vi "Generic IED Test.vi"(8 "error in":errorcluster, 11 "IED Test in":refnum<class "IED Test.lvclass">) -> (0 "error out":errorcluster, 2 "Test Result":T1=enum."Success", 3 "IED Test out":refnum<class "IED Test.lvclass">)   [LabVIEW 2018, in "IED Test Framework.lvlib" / "IED Test.lvclass"]
uses:
  IED Test.lvclass
  C:/Program Files (x86)/National Instruments/LabVIEW 2018/vi.lib/ActorFramework/Actor/Actor.lvclass
  C:/Users/Administrator/Desktop/2018LabVIEW EMS/EMS Generic Actor/EMS Generic/EMS Generic.lvclass
  Controls/Test Result.ctl
  IED Actor/IED/IED.lvclass
  C:/Users/Administrator/Desktop/2018LabVIEW EMS/IED Actors/Device DDS Communications Framework/Device DDS Communications/Device DDS Communications.lvclass
  <vilib>/ORNL/CSEISMIC DDS/CSEISMIC DDS Base/Data Types/Controls/DeviceClass Selector.ctl
  <vilib>/ORNL/CSEISMIC DDS/CSEISMIC DDS Base/CSEISMIC DDS.lvclass/CSEISMIC DDS.ctl
  <vilib>/ActorFramework/Message Enqueuer/Message Enqueuer.lvclass/Message Enqueuer.ctl
  <vilib>/ORNL/CSEISMIC DDS/CSEISMIC DDS Base/Data Types/Controls/DeviceID.ctl
  <vilib>/ORNL/CSEISMIC DDS/CSEISMIC DDS Base/Accessors/Write DDS Reference.vi
  <vilib>/ActorFramework/Message Enqueuer/Enqueue.vi
  <vilib>/ORNL/CSEISMIC DDS/CSEISMIC DDS Base/Accessors/Read DDS Reference.vi
  <vilib>/ORNL/CSEISMIC DDS/DDS Reader/DDS Reader.lvclass
  C:/Program Files (x86)/National Instruments/LabVIEW 2018/vi.lib/ORNL/CSEISMIC DDS/CSEISMIC DDS Base/CSEISMIC DDS.lvclass
  IED Actor/IED Messages/Set Microgrid ID Msg/Set Microgrid ID Msg.lvclass
  C:/Program Files (x86)/National Instruments/LabVIEW 2018/vi.lib/ActorFramework/Message/Message.lvclass
  <vilib>/ORNL/CSEISMIC DDS/DDS Writer/DDS Writer.lvclass
  <vilib>/ActorFramework/Stop Msg/Stop Msg.lvclass
  <vilib>/ORNL/CSEISMIC DDS/CSEISMIC DDS Base/Error Handler.vi
  <vilib>/ActorFramework/Message Priority Queue/Priority Enqueue.vi
  Device DDS Communications Framework/Device DDS Communications/Device DDS Communications.lvclass
  <vilib>/ActorFramework/Actor/Actor.lvclass
  <vilib>/ORNL/CSEISMIC DDS/CSEISMIC DDS Base/CSEISMIC DDS.lvclass
  EMS Generic Actor/EMS Generic/EMS Generic.lvclass
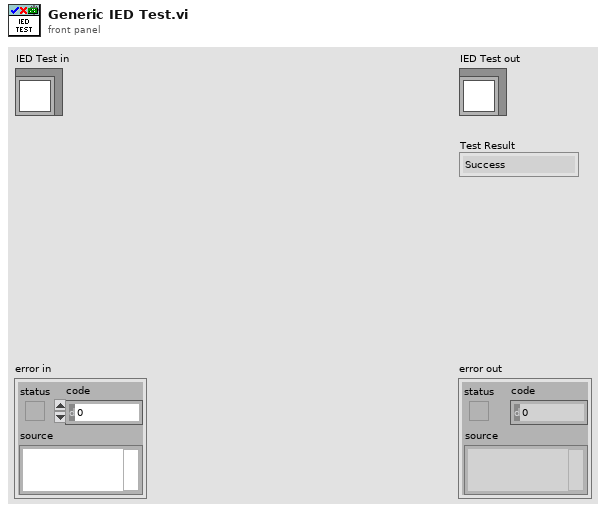
[diagram p1: front panel]
types:
  T1 = typedef "IED Test Framework.lvlib/IED Test.lvclass/Test Result.ctl" = enum16{"Invalid", "Success", "Failure", "Error", "Timeout"}
  T2 = typedef "CSEISMIC DDS.lvlib/CSEISMIC DDS.lvclass/DeviceID.ctl" = string
  T3 = typedef "CSEISMIC DDS.lvlib/CSEISMIC DDS.lvclass/DeviceClass Selector.ctl" = u16
  T4 = typedef "CSEISMIC DDS.lvlib/CSEISMIC DDS.lvclass/IED_setMicrogridID.ctl" = cluster{"DeviceID":T2, "MicrogridID":u8}
  T5 = typedef "CSEISMIC DDS.lvlib/CSEISMIC DDS.lvclass/IED_Status.ctl" = cluster{"DeviceID":T2, "Timestamp":T6, "MicrogridID":u8, "Active":bool, "Inactive":bool, "Error":i32, "Fault":bool, "ErrorString":string}
  T6 = typedef "CSEISMIC DDS.lvlib/CSEISMIC DDS.lvclass/Timestamp.ctl" = cluster{"Seconds":u64, "Remainder":u64}
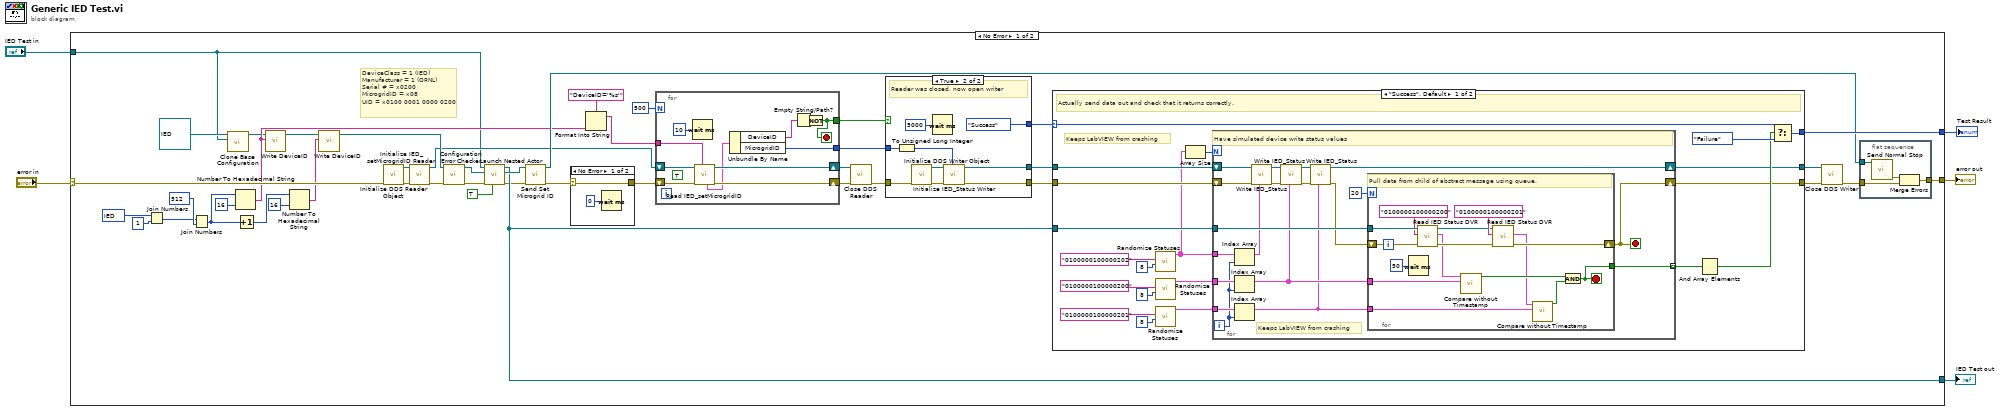
[diagram p0: block diagram]
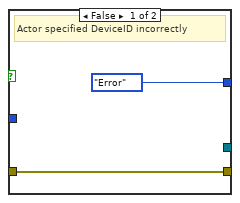
[diagram p3: hidden frame]
diagram:
  n1 = case shown="No Error" "error in" {
    selector: "error in" -> [w27 w138]
    tunnel: [w34 w138] -> w4
    tunnel: [w40 w137] -> w2
    tunnel: "IED Test in" -> [w6 w137]
    tunnel: [w37 _] -> w1
    frame No Error {
      w28 = T3 256 items=["Invalid"=0, "IED"=256, "DER"=512, "Relay"=768, "Meter"=1024, "Load"=1280, "Forecast"=1536, "Price"=1792, "Energy Storage"=513, "PV"=514, "Generator"=515, "Smart Relay"=769, "PCC"=770, "Smart Meter"=1025, "PMU"=1026, "HVAC"=1281] ("DeviceClass")
      # "DeviceClass = 1 (IED)\nManufacturer = 1 (ORNL)\nSerial # = x0200\nMicrogridID = x08\nUID = x0100 0001 0000 0200"
      n2 = Join Numbers(hi=w28, lo=u16 1 ("MicrogridID")) -> ((hi.lo)=w45:u32)
      n3 = Join Numbers(hi=w45, lo=u32 512 ("MicrogridID")) -> ((hi.lo)=w18:u64)
      n4 = call-dynamic "Clone Base Configuration.vi"("Source Object"=w6, "Target Object in"=refnum<class "IED.lvclass"> refnum ("IED Framework.lvlib:IED.lvclass")) -> ("Target Object out"=w7:refnum<class "IED.lvclass">)  [unwired: 9 in]
      n5 = Number To Hexadecimal String(1:i16 16 ("width (-)"), 2:w18) -> (0:w10:string)
      n6 = Increment(x=w18) -> (x+1=w16:u64)
      n7 = call-dynamic "Write DeviceID.vi"("DeviceID"=w10, "Device DDS Communications in"=w7) -> ("Device DDS Communications out"=w36:refnum<class "IED.lvclass">)  [unwired: 9 in]
      n8 = Number To Hexadecimal String(1:i16 16 ("width (-)"), 2:w16) -> (0:w15:string)
      n9 = call-dynamic "Write DeviceID.vi"("DeviceID"=w15, "Device DDS Communications in"=w36) -> ("Device DDS Communications out"=w35:refnum<class "IED.lvclass">)  [unwired: 9 in]
      n10 = call <vilib>:"Initialize DDS Reader Object.vi"("error in"=w27) -> ("error out"=w26:errorcluster, "DDS Reader out"=w25:refnum<class "DDS Reader.lvclass">)  [unwired: 9 in]
      n11 = call <vilib>:"Initialize IED_setMicrogridID Reader.vi"("error in"=w26, "DDS Reader in"=w25) -> ("error out"=w24:errorcluster, "DDS Reader out"=w23:refnum<class "DDS Reader.lvclass">)  [unwired: 8 in]
      n12 = call "Configuration Error Checker.vi"("error in"=w24, "Device DDS Communications in"=w35) -> ("error out"=w48:errorcluster, "Device DDS Communications out"=w47:refnum<class "IED.lvclass">)  [unwired: 8 in]
      n13 = call <vilib>:"Launch Nested Actor.vi"("Open Actor Core front panel? (F)"=TRUE, "error in (no error)"=w48, "Nested Actor"=w47, "Caller Actor in"=w6) -> ("error out"=w31:errorcluster, "Nested Actor's Enqueuer"=w49:refnum<class "Message Enqueuer.lvclass">, "Caller Actor out"=w40:refnum<class "IED Test.lvclass">)  [unwired: 5 in]
      n14 = call "Send Set Microgrid ID.vi"("error in (no error)"=w31, "Message Enqueuer"=w49) -> ("error out"=w30:errorcluster, "Message Enqueuer out"=w33:refnum<class "Message Enqueuer.lvclass">)  [unwired: 8 in]
      n15 = case shown="No Error" w30 {
        selector: w30 -> [w134 w136]
        tunnel: [w134 w136] -> w29
        frame No Error {
          n16 = Wait (ms)(milliseconds to wait=u32 0) -> ()  [unwired: 1 out]
        }
        frame Error {
        }
      }
      n17 = Format Into String(format string="DeviceID='%s'", w10) -> (resulting string=w9:string)  [unwired: 2 in, 1 out]
      n18 = for {
        N: 500 -> [_]
        tunnel: [w122] -> w43
        tunnel: [w118] -> w42
        shift-right: [w114] -> w21
        shift-left: w23 -> [w117]
        shift-right: [w115] -> w22
        shift-left: w29 -> [w116]
        tunnel: w9 -> [w112]
        stop <- w118 stop-if-true
        (unwired) TRUE ("only new samples")
        n19 = Wait (ms)(milliseconds to wait=u32 10) -> ()  [unwired: 1 out]
        n20 = call <vilib>:"Read IED_setMicrogridID.vi"("Query condition"=w112, "error in"=w116, "DDS Reader in"=w117) -> ("error out"=w115:errorcluster, "DDS Reader out"=w114:refnum<class "DDS Reader.lvclass">, "data"=w113:T4)  [unwired: 5 in, 1 out]
        n21 = Unbundle By Name(w113) -> ("DeviceID"=w121:T2, "MicrogridID"=w122:u8)
        n22 = Empty String/Path?(string/path=w121) -> (empty?=w119:bool)
        n23 = Not(x=w119) -> (.not. x?=w118:bool)
      }
      n24 = call <vilib>:"Close DDS Reader.vi"("error in"=w22, "DDS Reader in"=w21) -> ("error out"=w20:errorcluster)  [unwired: 9 in]
      n25 = case shown="True" w42 {
        tunnel: [w124 w128] -> w39
        tunnel: w20 -> [w124 w130]
        tunnel: w43 -> [_ w133]
        tunnel: [_ w125] -> w41
        tunnel: [Test_Result."Error" ("Test Result") Test_Result."Success" ("Test Result")] -> w38
        frame False {
          # "Actor specified DeviceID incorrectly"
        }
        frame True {
          # "Reader was closed, now open writer"
          n26 = To Unsigned Long Integer(number=w133) -> (unsigned 32bit integer=w126:u32)
          n27 = call <vilib>:"Initialize DDS Writer Object.vi"("error in"=w130) -> ("error out"=w129:errorcluster, "DDS Writer out"=w127:refnum<class "DDS Writer.lvclass">)  [unwired: 9 in]
          n28 = Wait (ms)(milliseconds to wait=u32 5000) -> ()  [unwired: 1 out]
          n29 = call <vilib>:"Initialize IED_Status Writer.vi"("MicrogridID"=w126, "error in"=w129, "DDS Writer in"=w127) -> ("error out"=w128:errorcluster, "DDS Writer out"=w125:refnum<class "DDS Writer.lvclass">)  [unwired: 7 in]
        }
      }
      n30 = case shown="\"Success\", Default" w38 {
        selector: w38 -> [w73 w110]
        tunnel: w41 -> [w74 w109]
        tunnel: w40 -> [w60 _]
        tunnel: w39 -> [w61 w111]
        tunnel: [w71 w110] -> w37
        tunnel: [w59 w111] -> w14
        tunnel: [w55 w109] -> w12
        frame "Success", Default {
          # "Keeps LabVIEW from crashing"
          # "Actually send data out and check that it returns correctly."
          n31 = call "Randomize Statuses.vi"("MicrogridID"=u16 8, "DeviceID"=T2 "0100000100000202" ("(hi.lo)")) -> ("IED Status Array out"=w56:T5[])  [unwired: 9 in]
          n32 = call "Randomize Statuses.vi"("MicrogridID"=u16 8, "DeviceID"=T2 "0100000100000200" ("(hi.lo)")) -> ("IED Status Array out"=w62:T5[])  [unwired: 9 in]
          n33 = call "Randomize Statuses.vi"("MicrogridID"=u16 8, "DeviceID"=T2 "0100000100000201" ("(hi.lo)")) -> ("IED Status Array out"=w63:T5[])  [unwired: 9 in]
          n34 = Array Size(array=w56) -> (size(s)=w57:i32)
          n35 = for {
            N: w57 -> [_]
            shift-right: [w90] -> w55
            shift-left: w74 -> [w93]
            tunnel: w56 -> [w86]
            tunnel: w63 -> [w81]
            tunnel: w62 -> [w82]
            shift-right: [w83] -> w59
            shift-left: w61 -> [w89]
            tunnel: w60 -> [w85]
            tunnel: [w75] -> w58 mode=indexing
            i -> [w78]
            stop <- w83 stop-if-true
            # "Keeps LabVIEW from crashing"
            # "Have simulated device write status values"
            n36 = Index Array(array=w86, index=w78) -> (element=w79:T5)
            n37 = Index Array(array=w82, index=w78) -> (element=w77:T5)
            n38 = Index Array(array=w81, index=w78) -> (element=w76:T5)
            n39 = call <vilib>:"Write IED_Status.vi"("IED_Status"=w79, "error in"=w89, "DDS Writer in"=w93) -> ("error out"=w88:errorcluster, "DDS Writer out"=w92:refnum<class "DDS Writer.lvclass">)  [unwired: 7 in]
            n40 = call <vilib>:"Write IED_Status.vi"("IED_Status"=w77, "error in"=w88, "DDS Writer in"=w92) -> ("error out"=w87:errorcluster, "DDS Writer out"=w91:refnum<class "DDS Writer.lvclass">)  [unwired: 7 in]
            n41 = call <vilib>:"Write IED_Status.vi"("IED_Status"=w76, "error in"=w87, "DDS Writer in"=w91) -> ("error out"=w84:errorcluster, "DDS Writer out"=w90:refnum<class "DDS Writer.lvclass">)  [unwired: 7 in]
            n42 = for {
              N: 20 -> [_]
              shift-right: [w102] -> w83
              shift-left: w84 -> [w108]
              tunnel: w85 -> [w107]
              tunnel: w77 -> [w101]
              tunnel: w76 -> [w94]
              tunnel: [w98] -> w75
              stop <- w98 stop-if-true
              # "Pull data from child of abstract message using queue."
              n43 = Wait (ms)(milliseconds to wait=u32 50) -> ()  [unwired: 1 out]
              n44 = call "Read IED Status DVR.vi"("error in"=w108, "DeviceID"=T2 "0100000100000200" ("(hi.lo)"), "EMS Generic in"=w107) -> ("error out"=w104:errorcluster, "IED_Status"=w100:T5, "EMS Generic out"=w103:refnum<class "IED Test.lvclass">)  [unwired: 5 in, 1 out]
              n45 = call "Compare without Timestamp.vi"("Status_IED gold"=w101, "IED_Status test"=w100) -> ("Boolean"=w99:bool)  [unwired: 9 in]
              n46 = call "Read IED Status DVR.vi"("error in"=w104, "DeviceID"=T2 "0100000100000201" ("(hi.lo)"), "EMS Generic in"=w103) -> ("error out"=w102:errorcluster, "IED_Status"=w95:T5)  [unwired: 5 in, 2 out]
              n47 = call "Compare without Timestamp.vi"("Status_IED gold"=w94, "IED_Status test"=w95) -> ("Boolean"=w96:bool)  [unwired: 9 in]
              n48 = And(x=w99, y=w96) -> (x .and. y?=w98:bool)
            }
          }
          n49 = And Array Elements(Boolean array=w58) -> (logical AND=w66:bool)
          n50 = Select(t=w73, s=w66, f=Test_Result."Failure") -> (s? t:f=w71:T1)
        }
        frame "Error" {
        }
      }
      n51 = call <vilib>:"Close DDS Writer.vi"("error in"=w14, "DDS Writer in"=w12) -> ("error out"=w13:errorcluster)  [unwired: 9 in]
      n52 = flat-sequence {
        tunnel: w33 -> [w54]
        tunnel: [w52] -> w34
        tunnel: w13 -> [w51]
        frame #0 {
          n53 = call <vilib>:"Send Normal Stop.vi"("Message Enqueuer"=w54) -> ("error out"=w53:errorcluster)  [unwired: 10 in]
          n54 = Merge Errors(w53, w51) -> (w52:errorcluster)
        }
      }
    }
    frame Error {
    }
  }
  "error out" <- w4
  "IED Test out" <- w2
  "Test Result" <- w1
